vi "get_ID.vi"(8 "error in (no error)":errorcluster, 11 "Agilent 34980A in":refnum<class "Agilent 34980A.lvclass">) -> (0 "error out":errorcluster, 2 "ID from instrument":string, 3 "Agilent 34980A out":refnum<class "Agilent 34980A.lvclass">)   [LabVIEW 2017, in "Agilent 34980A.lvclass"]
uses:
  Agilent 34980A.lvclass
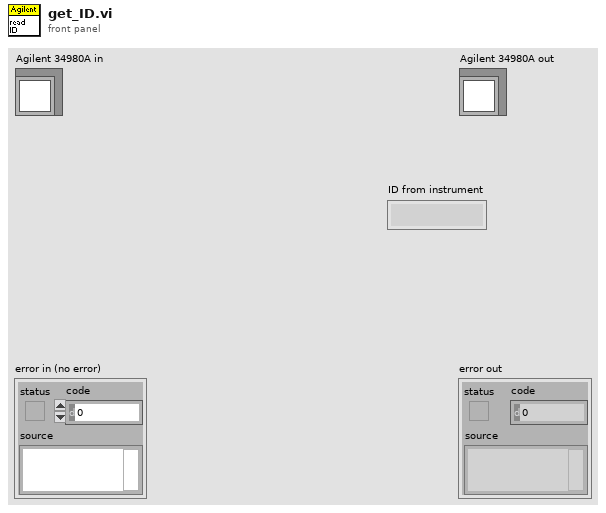
[diagram p1: front panel]
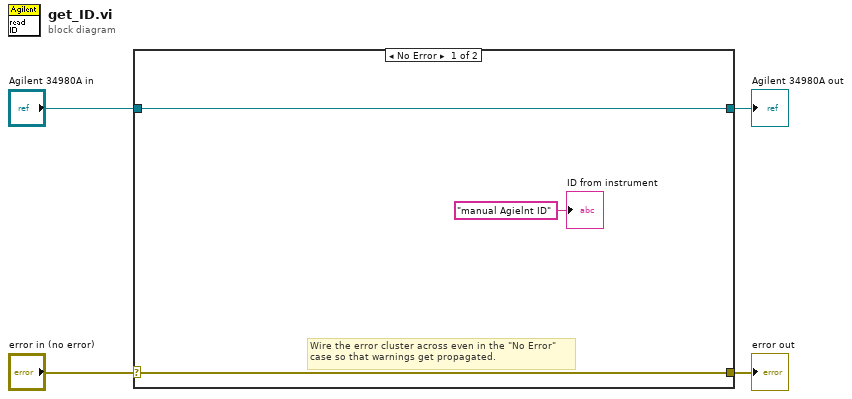
[diagram p0: block diagram]
diagram:
  n1 = case shown="No Error" "error in (no error)" {
    selector: "error in (no error)" -> [w6 w9]
    tunnel: [w6 w9] -> w3
    tunnel: [w7 w8] -> w1
    tunnel: "Agilent 34980A in" -> [w7 w8]
    frame No Error {
      # "Wire the error cluster across even in the \"No Error\"\ncase so that warnings get propagated."
      "ID from instrument" <- "manual Agielnt ID" ("ID from instrument")
    }
    frame Error {
    }
  }
  "error out" <- w3
  "Agilent 34980A out" <- w1
